vi "ClimberHome.vi"(0 "Home Start":bool, 1 "Front Climb Motor DevRef":T1={"DeviceStatus"={"status"=FALSE, "code"=0, "source"=""}, "Type"=enum."PWM", "PWM"={"PWM Channel"=enum."Invalid", "DeadBand"={"Name"="", "maxPositivePwm"=0, "minPositivePwm"=0, "centerPwm"=0, "maxNegativePwm"=0, "minNegativePwm"=0, "angularRange"=0}}, "CAN"={"Device Number"=0, "SetOutput VI Ref"=variant(enum8{"Percent VBus", "Current", "Speed", "Position", "Voltage"} enum."Percent VBus"), "GetOutput VI Ref"=variant(refnum<k1> refnum), "Enable VI Ref"=variant(dbl 12.0), "Disable VI Ref"=variant(enum8{"Percent VBus", "Speed", "Position", "Slave", "Unchanged / Invalid", "Voltage Compensation", "Current", "Motion Profile"} enum."Percent VBus"), "Data"=variant}, "Invert"=FALSE, "DIO PWM"={"PWM \"Enable\" Channel"=enum."Invalid", "DIOChannel"=enum."Invalid", "PWM Rate"=0.0}}, 2 "Home Invalidate":bool, 3 "Reset":bool, 4 "Back Climb Motor DevRef":T1={"DeviceStatus"={"status"=FALSE, "code"=0, "source"=""}, "Type"=enum."PWM", "PWM"={"PWM Channel"=enum."Invalid", "DeadBand"={"Name"="", "maxPositivePwm"=0, "minPositivePwm"=0, "centerPwm"=0, "maxNegativePwm"=0, "minNegativePwm"=0, "angularRange"=0}}, "CAN"={"Device Number"=0, "SetOutput VI Ref"=variant(enum8{"Percent VBus", "Current", "Speed", "Position", "Voltage"} enum."Percent VBus"), "GetOutput VI Ref"=variant(refnum<k1> refnum), "Enable VI Ref"=variant(dbl 12.0), "Disable VI Ref"=variant(enum8{"Percent VBus", "Speed", "Position", "Slave", "Unchanged / Invalid", "Voltage Compensation", "Current", "Motion Profile"} enum."Percent VBus"), "Data"=variant}, "Invert"=FALSE, "DIO PWM"={"PWM \"Enable\" Channel"=enum."Invalid", "DIOChannel"=enum."Invalid", "PWM Rate"=0.0}}, 5 "RobotConfig":T7={"Motors"={"DriveRightPrimary"={"CAN Address"=1, "Invert"=FALSE, "InvertSensor"=FALSE, "Unit Conversion Factor"=0.0, "Brake Mode"=enum."Override to Brake", "Reverse Limt Switch Mode"=enum."Normally Closed", "Forward Limt Swith Mode"=enum."Normally Closed", "PWM Channel"=enum."Invalid", "Motor Controller Type"=enum."Talon SRX", "Peak Current (A)"=0, "Continuos Current (A)"=0, "Peak Duration (ms)"=0, "Current Limit Enable"=FALSE}, "DriveRightSecondary"={"CAN Address"=2, "Invert"=FALSE, "InvertSensor"=FALSE, "Unit Conversion Factor"=0.0, "Brake Mode"=enum."Override to Brake", "Reverse Limt Switch Mode"=enum."Normally Closed", "Forward Limt Swith Mode"=enum."Normally Closed", "PWM Channel"=enum."Invalid", "Motor Controller Type"=enum."Talon SRX", "Peak Current (A)"=0, "Continuos Current (A)"=0, "Peak Duration (ms)"=0, "Current Limit Enable"=FALSE}, "DriveLeftPrimary"={"CAN Address"=3, "Invert"=FALSE, "InvertSensor"=FALSE, "Unit Conversion Factor"=0.0, "Brake Mode"=enum."Override to Brake", "Reverse Limt Switch Mode"=enum."Normally Closed", "Forward Limt Swith Mode"=enum."Normally Closed", "PWM Channel"=enum."Invalid", "Motor Controller Type"=enum."Talon SRX", "Peak Current (A)"=0, "Continuos Current (A)"=0, "Peak Duration (ms)"=0, "Current Limit Enable"=FALSE}, "DriveLeftSecondary"={"CAN Address"=4, "Invert"=FALSE, "InvertSensor"=FALSE, "Unit Conversion Factor"=0.0, "Brake Mode"=enum."Override to Brake", "Reverse Limt Switch Mode"=enum."Normally Closed", "Forward Limt Swith Mode"=enum."Normally Closed", "PWM Channel"=enum."Invalid", "Motor Controller Type"=enum."Talon SRX", "Peak Current (A)"=0, "Continuos Current (A)"=0, "Peak Duration (ms)"=0, "Current Limit Enable"=FALSE}, "RearClimb"={"CAN Address"=8, "Invert"=FALSE, "InvertSensor"=FALSE, "Unit Conversion Factor"=0.0, "Brake Mode"=enum."Override to Brake", "Reverse Limt Switch Mode"=enum."Normally Closed", "Forward Limt Swith Mode"=enum."Normally Closed", "PWM Channel"=enum."Invalid", "Motor Controller Type"=enum."Talon SRX", "Peak Current (A)"=0, "Continuos Current (A)"=0, "Peak Duration (ms)"=0, "Current Limit Enable"=FALSE}, "Front Climb"={"CAN Address"=7, "Invert"=FALSE, "InvertSensor"=FALSE, "Unit Conversion Factor"=0.0, "Brake Mode"=enum."Override to Brake", "Reverse Limt Switch Mode"=enum."Normally Closed", "Forward Limt Swith Mode"=enum."Normally Closed", "PWM Channel"=enum."Invalid", "Motor Controller Type"=enum."Talon SRX", "Peak Current (A)"=0, "Continuos Current (A)"=0, "Peak Duration (ms)"=0, "Current Limit Enable"=FALSE}, "Climb Drive"={"CAN Address"=5, "Invert"=FALSE, "InvertSensor"=FALSE, "Unit Conversion Factor"=0.0, "Brake Mode"=enum."Override to Brake", "Reverse Limt Switch Mode"=enum."Normally Closed", "Forward Limt Swith Mode"=enum."Normally Closed", "PWM Channel"=enum."Invalid", "Motor Controller Type"=enum."Talon SRX", "Peak Current (A)"=0, "Continuos Current (A)"=0, "Peak Duration (ms)"=0, "Current Limit Enable"=FALSE}, "Shoulder1"={"CAN Address"=6, "Invert"=FALSE, "InvertSensor"=FALSE, "Unit Conversion Factor"=0.0, "Brake Mode"=enum."Override to Brake", "Reverse Limt Switch Mode"=enum."Normally Closed", "Forward Limt Swith Mode"=enum."Normally Closed", "PWM Channel"=enum."Invalid", "Motor Controller Type"=enum."Talon SRX", "Peak Current (A)"=0, "Continuos Current (A)"=0, "Peak Duration (ms)"=0, "Current Limit Enable"=FALSE}, "Shoulder2"={"CAN Address"=9, "Invert"=FALSE, "InvertSensor"=FALSE, "Unit Conversion Factor"=0.0, "Brake Mode"=enum."Override to Brake", "Reverse Limt Switch Mode"=enum."Normally Closed", "Forward Limt Swith Mode"=enum."Normally Closed", "PWM Channel"=enum."Invalid", "Motor Controller Type"=enum."Talon SRX", "Peak Current (A)"=0, "Continuos Current (A)"=0, "Peak Duration (ms)"=0, "Current Limit Enable"=FALSE}, "Wrist"={"CAN Address"=10, "Invert"=FALSE, "InvertSensor"=FALSE, "Unit Conversion Factor"=0.0, "Brake Mode"=enum."Override to Brake", "Reverse Limt Switch Mode"=enum."Disabled", "Forward Limt Swith Mode"=enum."Disabled", "PWM Channel"=enum."Invalid", "Motor Controller Type"=enum."Talon SRX", "Peak Current (A)"=0, "Continuos Current (A)"=0, "Peak Duration (ms)"=0, "Current Limit Enable"=FALSE}, "Extension"={"CAN Address"=11, "Invert"=FALSE, "InvertSensor"=FALSE, "Unit Conversion Factor"=0.0, "Brake Mode"=enum."Override to Brake", "Reverse Limt Switch Mode"=enum."Disabled", "Forward Limt Swith Mode"=enum."Disabled", "PWM Channel"=enum."Invalid", "Motor Controller Type"=enum."Talon SRX", "Peak Current (A)"=0, "Continuos Current (A)"=0, "Peak Duration (ms)"=0, "Current Limit Enable"=FALSE}, "Intake1"={"CAN Address"=11, "Invert"=FALSE, "InvertSensor"=FALSE, "Unit Conversion Factor"=0.0, "Brake Mode"=enum."Override to Brake", "Reverse Limt Switch Mode"=enum."Disabled", "Forward Limt Swith Mode"=enum."Disabled", "PWM Channel"=enum."Invalid", "Motor Controller Type"=enum."Talon SRX", "Peak Current (A)"=0, "Continuos Current (A)"=0, "Peak Duration (ms)"=0, "Current Limit Enable"=FALSE}, "Intake2"={"CAN Address"=11, "Invert"=FALSE, "InvertSensor"=FALSE, "Unit Conversion Factor"=0.0, "Brake Mode"=enum."Override to Brake", "Reverse Limt Switch Mode"=enum."Disabled", "Forward Limt Swith Mode"=enum."Disabled", "PWM Channel"=enum."Invalid", "Motor Controller Type"=enum."Talon SRX", "Peak Current (A)"=0, "Continuos Current (A)"=0, "Peak Duration (ms)"=0, "Current Limit Enable"=FALSE}}, "Sensors"={"IMU"={"Yaw Axis"=enum."Z", "SPI Bus"=enum."SPI MXP", "AHRS Algorithm"=enum."Complementary", "Calibration Time (s)"=3.0, "Calibrate On Open"=TRUE}}, "PID"={"FrontClimb"={"P"=0.0, "I"=0.0, "D"=0.0, "F"=0.0, "IZone"=0.0}, "RearClimb"={"P"=0.0, "I"=0.0, "D"=0.0, "F"=0.0, "IZone"=0.0}, "ArmShoulder"={"P"=0.0, "I"=0.0, "D"=0.0, "F"=0.0, "IZone"=0.0}, "ArmExtend"={"P"=0.0, "I"=0.0, "D"=0.0, "F"=0.0, "IZone"=0.0}, "ArmWrist"={"P"=0.0, "I"=0.0, "D"=0.0, "F"=0.0, "IZone"=0.0}}, "Solenoids"={" Shifter"={"SolenoidChannel"=enum."Solenoid 3", "Invert"=FALSE}, "Hatch Grip"={"SolenoidChannel"=enum."Solenoid 0", "Invert"=FALSE}, "Hatch Extend"={"SolenoidChannel"=enum."Solenoid 0", "Invert"=FALSE}, "Manipulator Slide"={"SolenoidChannel"=enum."Solenoid 0", "Invert"=FALSE}, "Hatch Floor Intake"={"SolenoidChannel"=enum."Solenoid 0", "Invert"=FALSE}}, "Enable Compressor"=TRUE, "MotionMagic"={"FrontClimb"={"CruiseVelocity"=0, "Acceleration"=0}, "RearClimb"={"CruiseVelocity"=0, "Acceleration"=0}}, "RobotDimensions"={"Length (in)"=0.0, "Shoulder Height (in)"=0.0, "Frame Height (in)"=0.0, "Arm Center to Front of Robot (in)"=0.0, "Arm Min Extension (in)"=0.0, "Arm Max Extension (in)"=0.0}, "Arm Home Position"={"Radius (in)"=0.0, "ShoulderAngle (rad)"=0.0, "WristAngle (rad)"=0.0}, "Climb Home Position"={"Back Climb"=0.0, "Front Climb"=0.0}, "Climb Positions"={"Retract"=0.0, "Level 2"=0.0, "Level 3"=0.0}}) -> (6 "Front Climb Motor Speed":dbl format="%#_13g", 7 "Back Climb Motor Speed":dbl format="%#_13g", 8 "Climber Home State":T6)   [LabVIEW 2018]
uses:
  TypeDefs/ConfigComponents/Config_Robot.ctl
  ArgosLib/Config/ConfigComponents/TypeDefs/Config_Motor.ctl
  <vilib>/Rock Robotics/WPI/ThirdParty/Phoenix-LabVIEW/Motor Controller/Controls/CTRE_Phoenix_MotorControl_NeutralMode.ctl
  <vilib>/Rock Robotics/WPI/ThirdParty/Phoenix-LabVIEW/Motor Controller/Controls/CTRE_Phoenix_MotorControl_LimitSwitchNormal.ctl
  <vilib>/Rock Robotics/SystemInterfaces/DIO/FPGA_DIOPWMChannel.ctl
  ArgosLib/Config/ConfigComponents/TypeDefs/Config_MotorCtrlType.ctl
  ArgosLib/Config/ConfigComponents/TypeDefs/Config_IMU.ctl
  <vilib>/Rock Robotics/SystemInterfaces/spilib/spi_bus.ctl
  ArgosLib/Config/ConfigComponents/TypeDefs/Config_PIDParams.ctl
  ArgosLib/Config/ConfigComponents/TypeDefs/Config_SingleSolenoid.ctl
  <vilib>/Rock Robotics/WPI/Solenoid/WPI_SolenoidChannel.ctl
  ArgosLib/Config/ConfigComponents/TypeDefs/Config_MotionMagicParams.ctl
  TypeDefs/ConfigComponents/Config_Dimensions.ctl
  Arm/TypeDefs/ArmCoordinate.ctl
  TypeDefs/ClimberPositionHeights.ctl
  TypeDefs/ClimberHomingState.ctl
  <vilib>/Rock Robotics/WPI/MotorControl/WPI_MotorControlDeviceRef.ctl
  <vilib>/Rock Robotics/WPI/MotorControl/WPI_MotorControlType.ctl
  <vilib>/Rock Robotics/WPI/PWM/WPI_PWMDeadband.ctl
  <vilib>/Rock Robotics/SystemInterfaces/DIO/FPGA_DIOChannel.ctl
  <vilib>/Rock Robotics/WPI/ThirdParty/Phoenix-LabVIEW/Motor Controller/Get/CTRE_Phoenix_MotorController_GetSelectedSensorData.vi
  ArgosLib/ArgosLib.lvlib
panel:
  in  "Homing TimeOut (ms)":u32=1500
  in  "Homing Stall Time (ms)":u32=250
  in  "Homing Stall Speed (in/s)":dbl=2.0
  in  "Homing Motor Speed":dbl=-0.25
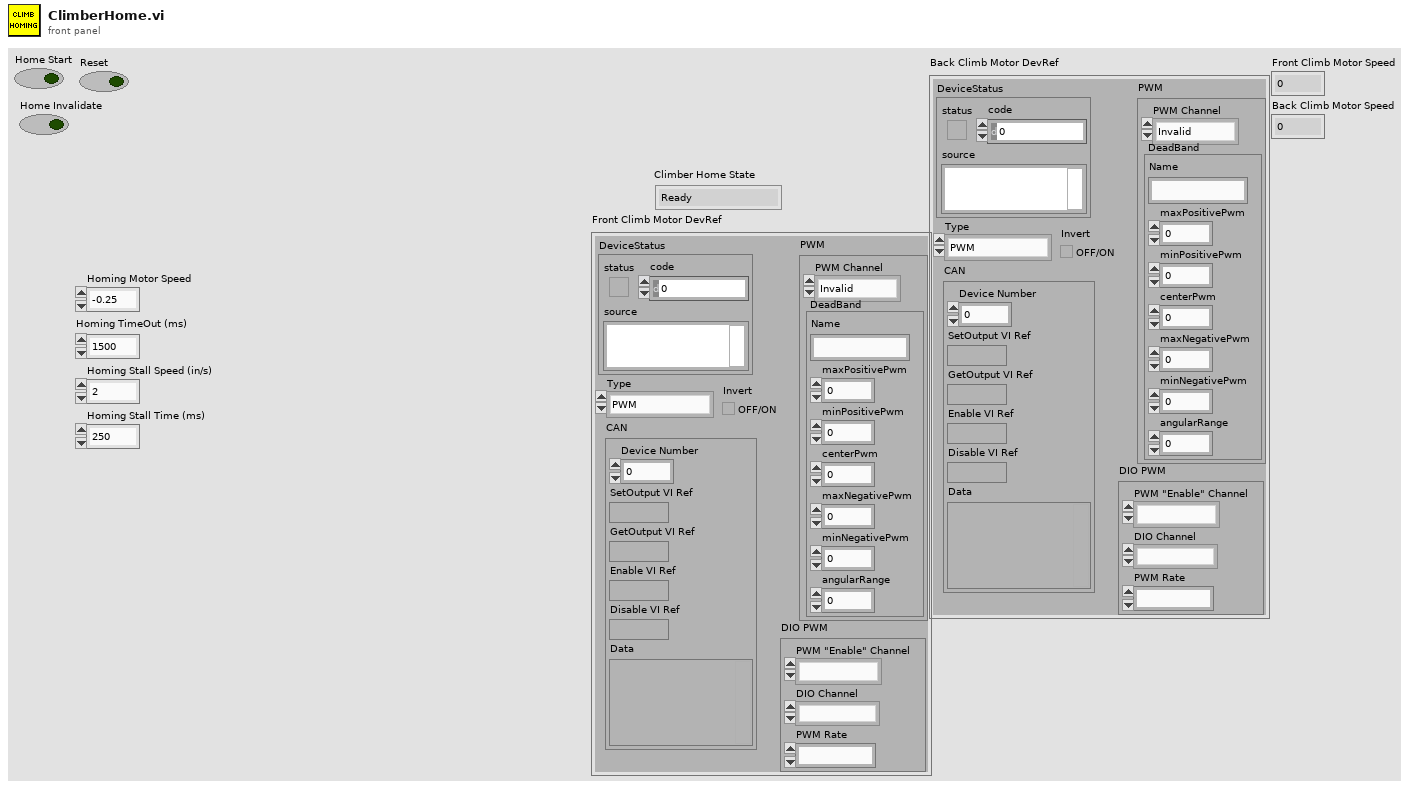
[diagram p1: front panel]
types:
  T1 = typedef "WPI_MotorControlDeviceRef.ctl" = cluster{"DeviceStatus":errorcluster, "Type":T2, "PWM":cluster{"PWM Channel":T3, "DeadBand":T4}, "CAN":cluster{"Device Number":u8, "SetOutput VI Ref":variant, "GetOutput VI Ref":variant, "Enable VI Ref":variant, "Disable VI Ref":variant, "Data":variant}, "Invert":bool, "DIO PWM":cluster{"PWM \"Enable\" Channel":T3, "DIOChannel":T5, "PWM Rate":dbl}}
  T2 = typedef "WPI_MotorControlType.ctl" = enum16{"PWM", "CAN", "DIO PWM"}
  T3 = typedef "FPGA_DIOPWMChannel.ctl" = enum8{"PWM 0", "PWM 1", "PWM 2", "PWM 3", "PWM 4", "PWM 5", "PWM 6", "PWM 7", "PWM 8", "PWM 9", "PWM MXP 0", "PWM MXP 1", "PWM MXP 2", "PWM MXP 3", "PWM MXP 4", "PWM MXP 5", "PWM MXP 6", "PWM MXP 7", "PWM MXP 8", "PWM MXP 9", "Invalid"}
  T4 = typedef "WPI_PWMDeadband.ctl" = cluster{"Name":string, "maxPositivePwm":i32, "minPositivePwm":i32, "centerPwm":i32, "maxNegativePwm":i32, "minNegativePwm":i32, "angularRange":u16}
  T5 = typedef "FPGA_DIOChannel.ctl" = enum8{"DIO 0", "DIO 1", "DIO 2", "DIO 3", "DIO 4", "DIO 5", "DIO 6", "DIO 7", "DIO 8", "DIO 9", "DIO MXP 0", "DIO MXP 1", "DIO MXP 2", "DIO MXP 3", "DIO MXP 4", "DIO MXP 5", "DIO MXP 6", "DIO MXP 7", "DIO MXP 8", "DIO MXP 9", "DIO MXP 10", "DIO MXP 11", "DIO MXP 12", "DIO MXP 13", "DIO MXP 14", "DIO MXP 15", "SPI Port CS1", "SPI Port CS2", "SPI Port CS3", "SPI Port MISO", "SPI Port MOSI", "Invalid"}
  T6 = typedef "ClimberHomingState.ctl" = enum16{"Ready", "Homing In progress", "Homing Failure", "Homing Success "}
  T7 = typedef "Config_Robot.ctl" = cluster{"Motors":cluster{"DriveRightPrimary":T8, "DriveRightSecondary":T8, "DriveLeftPrimary":T8, "DriveLeftSecondary":T8, "RearClimb":T8, "Front Climb":T8, "Climb Drive":T8, "Shoulder1":T8, "Shoulder2":T8, "Wrist":T8, "Extension":T8, "Intake1":T8, "Intake2":T8}, "Sensors":cluster{"IMU":T12}, "PID":cluster{"FrontClimb":T14, "RearClimb":T14, "ArmShoulder":T14, "ArmExtend":T14, "ArmWrist":T14}, "Solenoids":cluster{" Shifter":T15, "Hatch Grip":T15, "Hatch Extend":T15, "Manipulator Slide":T15, "Hatch Floor Intake":T15}, "Enable Compressor":bool, "MotionMagic":cluster{"FrontClimb":T17, "RearClimb":T17}, "RobotDimensions":T18, "Arm Home Position":T19, "Climb Home Position":cluster{"Back Climb":dbl, "Front Climb":dbl}, "Climb Positions":T20}
  T8 = typedef "ArgosLib.lvlib/Config_Motor.ctl" = cluster{"CAN Address":u8, "Invert":bool, "InvertSensor":bool, "Unit Conversion Factor":dbl, "Brake Mode":T9, "Reverse Limt Switch Mode":T10, "Forward Limt Swith Mode":T10, "PWM Channel":T3, "Motor Controller Type":T11, "Peak Current (A)":i32, "Continuos Current (A)":i32, "Peak Duration (ms)":i32, "Current Limit Enable":bool}
  T9 = typedef "CTRE_Phoenix_MotorControl_NeutralMode.ctl" = enum8{"EEPROMSetting", "Override to Coast", "Override to Brake"}
  T10 = typedef "CTRE_Phoenix_MotorControl_LimitSwitchNormal.ctl" = enum16{"Normally Open", "Normally Closed", "Disabled"}
  T11 = typedef "ArgosLib.lvlib/Config_MotorCtrlType.ctl" = enum16{"Disabled", "Talon SRX", "Talon SR"}
  T12 = typedef "ArgosLib.lvlib/Config_IMU.ctl" = cluster{"Yaw Axis":enum16{"X", "Y", "Z"}, "SPI Bus":T13, "AHRS Algorithm":enum16{"Complementary", "Madgwick"}, "Calibration Time (s)":dbl, "Calibrate On Open":bool}
  T13 = typedef "spi_bus.ctl" = enum16{"SPI On-Board, CS0", "SPI On-Board, CS1", "SPI On-Board, CS2", "SPI On-Board, CS3", "SPI MXP", "Invalid"}
  T14 = typedef "ArgosLib.lvlib/Config_PIDParams.ctl" = cluster{"P":dbl, "I":dbl, "D":dbl, "F":dbl, "IZone":dbl}
  T15 = typedef "ArgosLib.lvlib/Config_SingleSolenoid.ctl" = cluster{"SolenoidChannel":T16, "Invert":bool}
  T16 = typedef "WPI_SolenoidChannel.ctl" = enum8{"Solenoid 0", "Solenoid 1", "Solenoid 2", "Solenoid 3", "Solenoid 4", "Solenoid 5", "Solenoid 6", "Solenoid 7", "Invalid"}
  T17 = typedef "Config_MotionMagicParams.ctl" = cluster{"CruiseVelocity":i32, "Acceleration":i32}
  T18 = typedef "Config_Dimensions.ctl" = cluster{"Length (in)":dbl, "Shoulder Height (in)":dbl, "Frame Height (in)":dbl, "Arm Center to Front of Robot (in)":dbl, "Arm Min Extension (in)":dbl, "Arm Max Extension (in)":dbl}
  T19 = typedef "ArmCoordinate.ctl" = cluster{"Radius (in)":dbl, "ShoulderAngle (rad)":dbl, "WristAngle (rad)":dbl}
  T20 = typedef "ClimberPositionHeights.ctl" = cluster{"Retract":dbl, "Level 2":dbl, "Level 3":dbl}
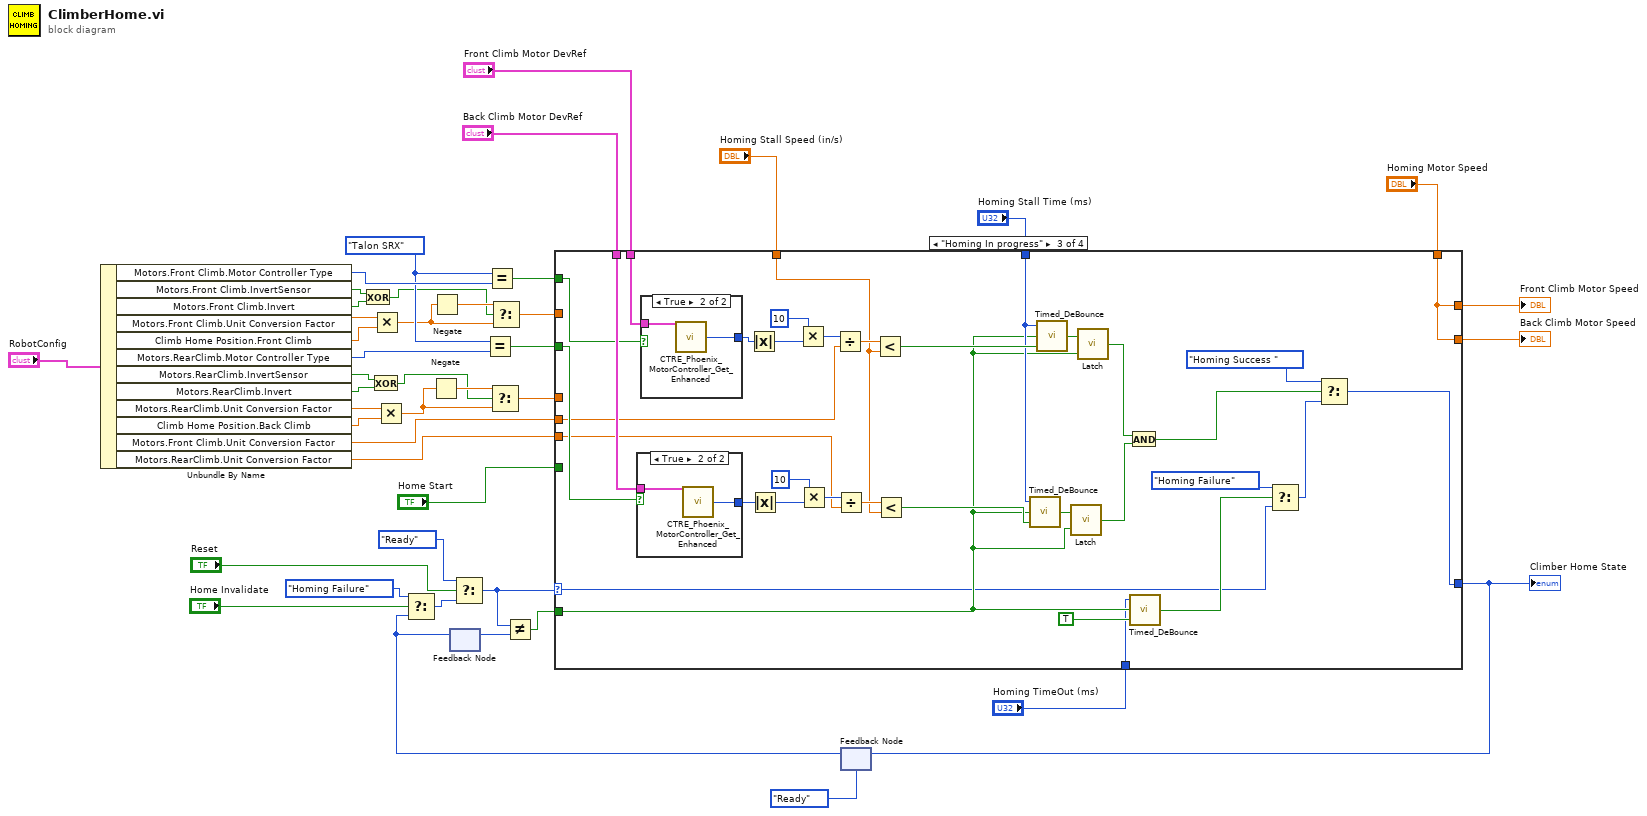
[diagram p0: block diagram]
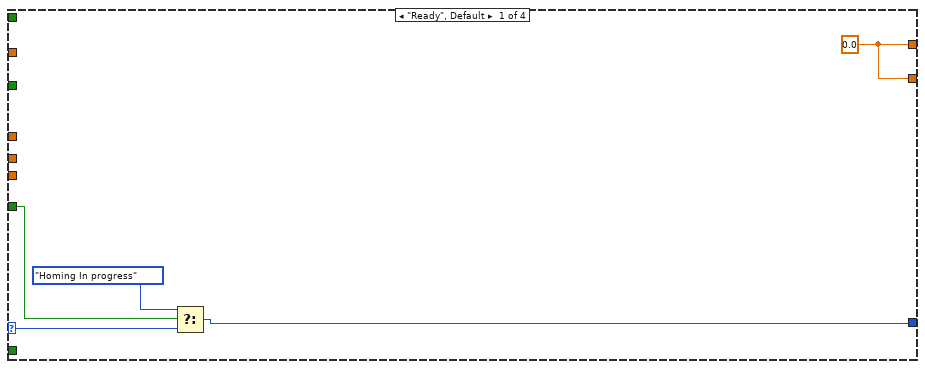
[diagram p2: hidden frame]
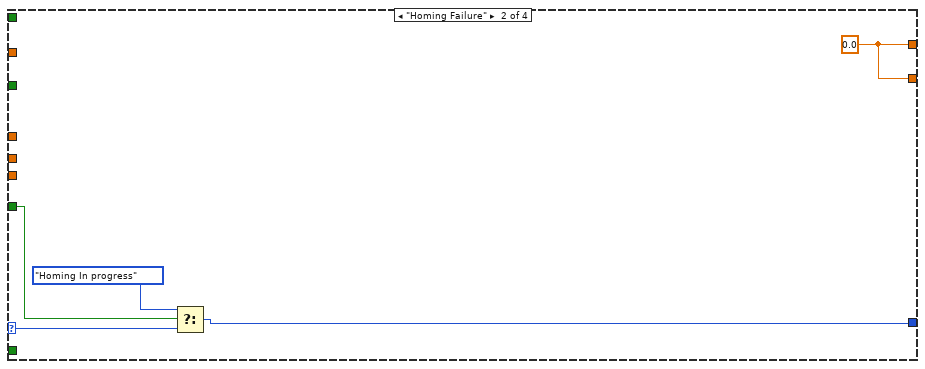
[diagram p3: hidden frame]
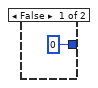
[diagram p4: hidden frame]
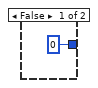
[diagram p5: hidden frame]
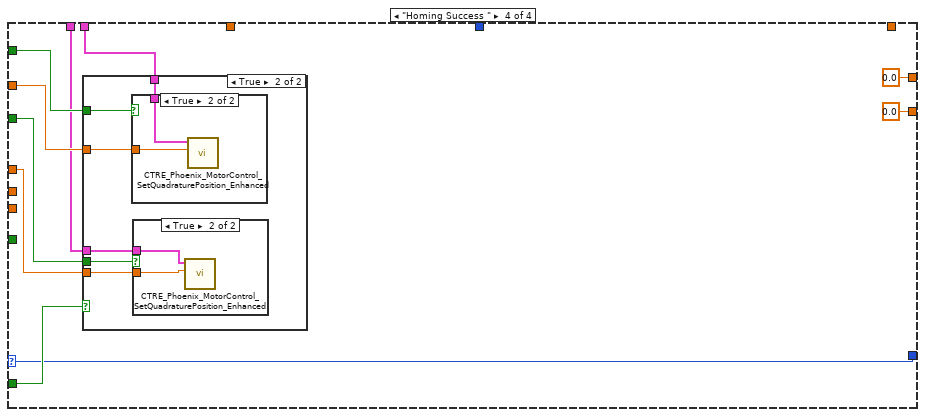
[diagram p6: hidden frame]
diagram:
  w34 = Config_MotorCtrlType."Talon SRX" ("x")
  n1 = Unbundle By Name("RobotConfig") -> ("Motors.Front Climb.Motor Controller Type"=w36:T11, "Motors.Front Climb.InvertSensor"=w5:bool, "Motors.Front Climb.Invert"=w6:bool, "Motors.Front Climb.Unit Conversion Factor"=w33:dbl, "Climb Home Position.Front Climb"=w32:dbl, "Motors.RearClimb.Motor Controller Type"=w35:T11, "Motors.RearClimb.InvertSensor"=w2:bool, "Motors.RearClimb.Invert"=w3:bool, "Motors.RearClimb.Unit Conversion Factor"=w29:dbl, "Climb Home Position.Back Climb"=w28:dbl, "Motors.Front Climb.Unit Conversion Factor"=w19:dbl, "Motors.RearClimb.Unit Conversion Factor"=w18:dbl)
  n2 = Exclusive Or(1:w6, 2:w5) -> (0:w4:bool)
  n3 = Exclusive Or(1:w3, 2:w2) -> (0:w1:bool)
  n4 = Multiply(x=w33, y=w32) -> (x*y=w30:dbl)
  n5 = Multiply(x=w29, y=w28) -> (x*y=w27:dbl)
  n6 = Negate(x=w27) -> (-x=w26:dbl)
  n7 = Negate(x=w30) -> (-x=w31:dbl)
  n8 = feedback #1() -> (w43:T6)  [unwired: 1 in]
  n9 = Equal?(x=w34, y=w35) -> (x = y?=w21:bool)
  n10 = Equal?(x=w34, y=w36) -> (x = y?=w23:bool)
  n11 = Select(t=w26, s=w1, f=w27) -> (s? t:f=w20:dbl)
  n12 = Select(t=w31, s=w4, f=w30) -> (s? t:f=w22:dbl)
  n13 = feedback #2(ClimberHomingState."Ready" ("Climber Home State")) -> (w14:T6)
  n14 = Select(t=ClimberHomingState."Homing Failure" ("Climber Home State"), s="Home Invalidate", f=w14) -> (s? t:f=w11:T6)
  n15 = feedback-in #1(w14) -> ()
  n16 = Select(t=ClimberHomingState."Ready" ("Climber Home State"), s="Reset", f=w11) -> (s? t:f=w7:T6)
  n17 = Not Equal?(x=w7, y=w43) -> (x != y?=w42:bool)
  n18 = case shown="\"Homing In progress\"" w7 {
    selector: w7 -> [w49 w54 w59 w98]
    tunnel: w42 -> [_ _ w63 w105]
    tunnel: "Home Start" -> [w48 w53 _ _]
    tunnel: [w46 w51 w55 w98] -> w10
    tunnel: [w45 w50 w89 0.0 ("Homing Motor Speed")] -> w40
    tunnel: [w45 w50 w89 0.0 ("Homing Motor Speed")] -> w39
    tunnel: "Homing Motor Speed" -> [_ _ w89 _]
    tunnel: "Front Climb Motor DevRef" -> [_ _ w88 w102]
    tunnel: "Back Climb Motor DevRef" -> [_ _ w87 w100]
    tunnel: w23 -> [_ _ w86 w104]
    tunnel: w22 -> [_ _ _ w101]
    tunnel: w21 -> [_ _ w85 w103]
    tunnel: w20 -> [_ _ _ w99]
    tunnel: w19 -> [_ _ w73 _]
    tunnel: w18 -> [_ _ w80 _]
    tunnel: "Homing Stall Speed (in/s)" -> [_ _ w72 _]
    tunnel: "Homing Stall Time (ms)" -> [_ _ w67 _]
    tunnel: "Homing TimeOut (ms)" -> [_ _ w62 _]
    frame "Ready", Default {
      w45 = 0.0 ("Front Climb Motor Speed")
      n19 = Select(t=ClimberHomingState."Homing In progress", s=w48, f=w49) -> (s? t:f=w46:T6)
    }
    frame "Homing Failure" {
      w50 = 0.0 ("Front Climb Motor Speed")
      n20 = Select(t=ClimberHomingState."Homing In progress", s=w53, f=w54) -> (s? t:f=w51:T6)
    }
    frame "Homing In progress" {
      n21 = case shown="True" w85 {
        tunnel: w87 -> [_ w92]
        tunnel: [0 ("Velocity (Raw Sensor Units per 100 ms)") w91] -> w84
        frame False {
        }
        frame True {
          n22 = call-poly <vilib>:"CTRE_Phoenix_MotorController_Get_Enhanced.vi"("PhoenixMotorControlDevRef"=w92) -> ("Velocity (Raw Sensor Units per 100 ms)"=w91:i32)  [unwired: 11 in, 3 out]
        }
      }
      n23 = case shown="True" w86 {
        tunnel: w88 -> [_ w95]
        tunnel: [0 ("Velocity (Raw Sensor Units per 100 ms)") w94] -> w74
        frame False {
        }
        frame True {
          n24 = call-poly <vilib>:"CTRE_Phoenix_MotorController_Get_Enhanced.vi"("PhoenixMotorControlDevRef"=w95) -> ("Velocity (Raw Sensor Units per 100 ms)"=w94:i32)  [unwired: 11 in, 3 out]
        }
      }
      n25 = Absolute Value(x=w74) -> (abs(x)=w78:i32)
      n26 = Absolute Value(x=w84) -> (abs(x)=w83:i32)
      n27 = Multiply(x=10, y=w78) -> (x*y=w76:i32)
      n28 = Multiply(x=10, y=w83) -> (x*y=w81:i32)
      n29 = Divide(x=w76, y=w73) -> (x/y=w75:dbl)
      n30 = Divide(x=w81, y=w80) -> (x/y=w79:dbl)
      n31 = Less?(x=w75, y=w72) -> (x < y?=w71:bool)
      n32 = Less?(x=w79, y=w72) -> (x < y?=w68:bool)
      n33 = call "Timed_DeBounce.vi"("Input"=w68, "Reset"=w63, "Hold Time(ms)"=w67) -> ("Output"=w69:bool)
      n34 = call "Timed_DeBounce.vi"("Input"=w71, "Reset"=w63, "Hold Time(ms)"=w67) -> ("Output"=w70:bool)
      n35 = call "Latch.vi"("Reset"=w63, "Input"=w69) -> ("LatchOut"=w65:bool)
      n36 = call "Latch.vi"("Reset"=w63, "Input"=w70) -> ("LatchOut"=w66:bool)
      n37 = And(x=w66, y=w65) -> (x .and. y?=w60:bool)
      n38 = call "Timed_DeBounce.vi"("Input"=TRUE, "Reset"=w63, "Hold Time(ms)"=w62) -> ("Output"=w61:bool)
      n39 = Select(t=ClimberHomingState."Homing Failure", s=w61, f=w59) -> (s? t:f=w57:T6)
      n40 = Select(t=ClimberHomingState."Homing Success ", s=w60, f=w57) -> (s? t:f=w55:T6)
    }
    frame "Homing Success " {
      n41 = case shown="True" w105 {
        tunnel: w104 -> [_ w111]
        tunnel: w103 -> [_ w110]
        tunnel: w102 -> [_ w109]
        tunnel: w101 -> [_ w108]
        tunnel: w100 -> [_ w107]
        tunnel: w99 -> [_ w106]
        frame False {
        }
        frame True {
          n42 = case shown="True" w111 {
            tunnel: w109 -> [_ w115]
            tunnel: w108 -> [_ w114]
            frame False {
            }
            frame True {
              n43 = call <vilib>:"CTRE_Phoenix_MotorControl_SetQuadraturePosition_Enhanced.vi"("New Position"=w114, "PhoenixMotorControlDevRef"=w115) -> ()  [unwired: 8 in, 2 out]
            }
          }
          n44 = case shown="True" w110 {
            tunnel: w107 -> [_ w113]
            tunnel: w106 -> [_ w112]
            frame False {
            }
            frame True {
              n45 = call <vilib>:"CTRE_Phoenix_MotorControl_SetQuadraturePosition_Enhanced.vi"("New Position"=w112, "PhoenixMotorControlDevRef"=w113) -> ()  [unwired: 8 in, 2 out]
            }
          }
        }
      }
    }
  }
  "Climber Home State" <- w10
  "Front Climb Motor Speed" <- w40
  "Back Climb Motor Speed" <- w39
  n46 = feedback-in #2(w10) -> ()
